vi "Add Roundkey.vi"(10 "Roundkey In":u8[](array[numeric])=[0, 0, 0, 0, 0, 0, 0, 0, 0, 0, 0, 0, 0, 0, 0, 0], 11 "Data In":u8[](array[numeric])=[0, 0, 0, 0, 0, 0, 0, 0, 0, 0, 0, 0, 0, 0, 0, 0]) -> (3 "Array Out":u8[](array[numeric]))   [LabVIEW 2017]
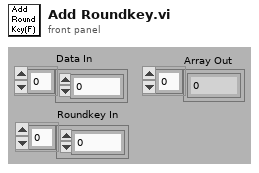
[diagram p1: front panel]
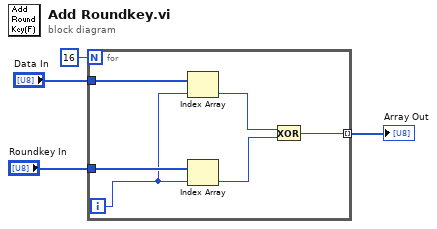
[diagram p0: block diagram]
diagram:
  n1 = for {
    N: 16 -> [_]
    tunnel: "Data In" -> [w10]
    tunnel: [w6] -> w3 mode=indexing
    tunnel: "Roundkey In" -> [w9]
    i -> [w5]
    n2 = Index Array(array=w10, index=w5) -> (element=w7:u8)
    n3 = Index Array(array=w9, index=w5) -> (element=w8:u8)
    n4 = Exclusive Or(1:w8, 2:w7) -> (0:w6:u8)
  }
  "Array Out" <- w3
